vi "RX Disabled channel logic 1ch 4SPC.vi"(7 "reset":bool, 9 "input valid":bool, 11 "U32 data in":u32[](array[numeric])=[0, 0, 0, 0]) -> (1 "data ready":bool, 3 "U32 data out":u32[](array[numeric]))   [LabVIEW 2025, in "niUSRP Stream Control (DMA) v1 FPGA.lvclass"]
uses:
  niUSRP Stream Control (DMA) v1 FPGA.lvclass
  niUSRP Stream Control (DMA) v1 FPGA.lvclass/niUSRP Stream Control (DMA) v1 FPGA.ctl
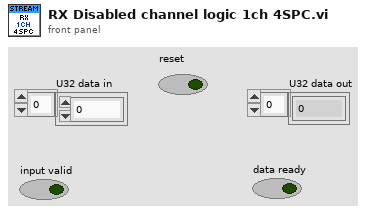
[diagram p1: front panel]
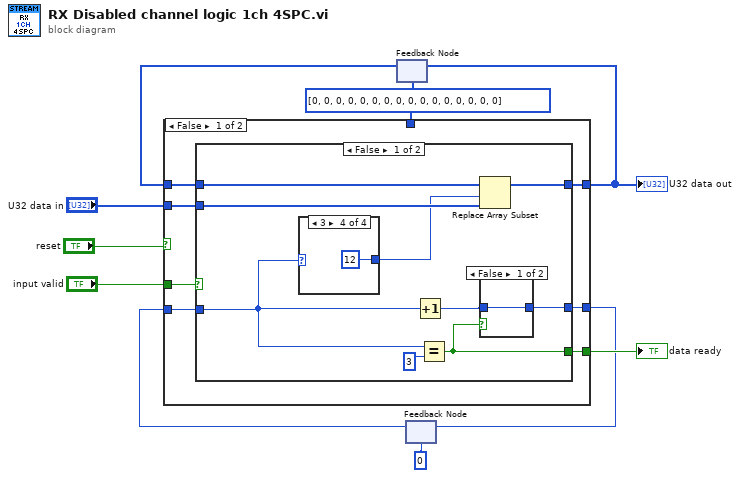
[diagram p0: block diagram]
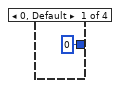
[diagram p2: hidden frame]
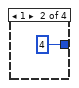
[diagram p3: hidden frame]
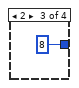
[diagram p4: hidden frame]
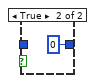
[diagram p5: hidden frame]
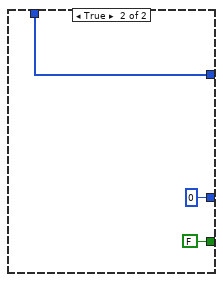
[diagram p7: hidden frame]
diagram:
  w1 = u32[] [0, 0, 0, 0, 0, 0, 0, 0, 0, 0, 0, 0, 0, 0, 0, 0]
  n1 = feedback #1(w1) -> (w5:u32[])
  n2 = feedback #2(u8 0) -> (w4:u8)
  n3 = case shown="False" "reset" {
    tunnel: [w17 FALSE] -> w10
    tunnel: [w16 u8 0] -> w9
    tunnel: [w15 w36] -> w8
    tunnel: "input valid" -> [w14 _]
    tunnel: "U32 data in" -> [w13 _]
    tunnel: w5 -> [w12 _]
    tunnel: w4 -> [w11 _]
    tunnel: w1 -> [_ w36]
    frame False {
      n4 = case shown="False" w14 {
        selector: w14 -> [_ w33]
        tunnel: w13 -> [w24 _]
        tunnel: w11 -> [w19 w35]
        tunnel: [w21 w35] -> w16
        tunnel: w12 -> [w26 w34]
        tunnel: [w25 w34] -> w15
        tunnel: [w22 w33] -> w17
        frame False {
          n5 = case shown="3" w19 {
            tunnel: [0 ("index") 4 ("index") 8 ("index") 12 ("index")] -> w18
            frame 0, Default {
            }
            frame 1 {
            }
            frame 2 {
            }
            frame 3 {
            }
          }
          n6 = Increment(x=w19) -> (x+1=w20:u8)
          n7 = Equal?(x=w19, y=u8 3) -> (x = y?=w22:bool)
          n8 = Replace Array Subset(array=w26, new element=w24, index=w18) -> (w25:u32[])
          n9 = case shown="False" w22 {
            tunnel: [w31 u8 0] -> w21
            tunnel: w20 -> [w31 _]
            frame False {
            }
            frame True {
            }
          }
        }
        frame True {
        }
      }
    }
    frame True {
    }
  }
  "data ready" <- w10
  "U32 data out" <- w8
  n10 = feedback-in #1(w8) -> ()
  n11 = feedback-in #2(w9) -> ()
